vi "Combine I&P.vi"() -> ()   [LabVIEW 2016]
uses:
  <vilib>/userdefined/High Color/IMAQdx.ctl
  <vilib>/vision/driver/NI_Vision_Acquisition_Software.lvlib
panel:
  out "Injector's Position":dbl[](array[numeric])
  in  "sutter run":bool
  in  "Refresh":bool
  out "Cells' pos":dbl[][](array[numeric])
  in  "Cell to Delete":dbl
  in  "stop capture":bool
  out "Image":T1(plugin-control)
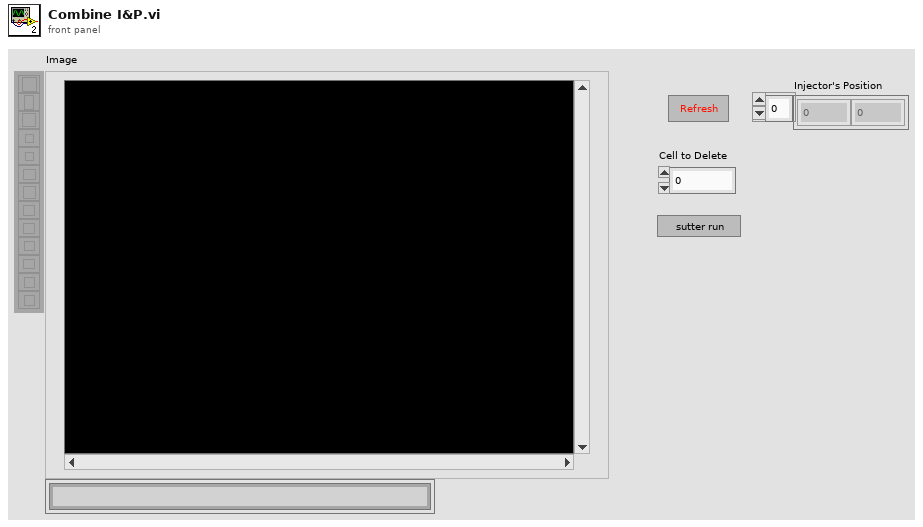
[diagram p1: front panel]
types:
  T1 = typedef "IMAQ Image.ctl" = refnum<image>
  T2 = typedef "IMAQdx.ctl" = refnum<k21>
  T3 = cluster{"Position":cluster{"x":sgl, "y":sgl}, "Angle":sgl, "Scale":sgl, "Score":sgl, "Bounding Box":cluster{"x":sgl, "y":sgl}[]}[]
  T4 = cluster{"Name":string, "Type":enum16{"Line", "Broken Line", "Free Hand Line", "Rotated Rectangle", "Oval", "Polygon", "Free Hand", "Bitmap", "Text"}, "Coordinates":i32[], "Colors":u32[], "Drawing Mode":u32, "Text":string, "Results":cluster{"Process ID":string, "Measure":u16, "Name":string, "String Format":u16, "Width":i16, "Precision":i16, "True String":string, "False String":string}[], "Font, Size & Style":cluster{"Desired Font (Application)":enum16{"User-specified Font", "Application Font", "System Font", "Dialog Font"}, "[User-specified Font]":cluster{"Font Name":string, "Size":i16, "Strikeout?":bool, "Italic?":bool, "Underline?":bool, "Outline?":bool, "Shadow?":bool, "Bold?":bool, "Rotation Angle":dbl}, "Horizontal Alignment":i16, "Vertical Alignment":i16}, "Image File Path":path, "Use Keying Color":bool}[]
  T5 = cluster{"Position":cluster{"x":sgl, "y":sgl}, "Angle":sgl, "Scale":sgl, "Score":sgl, "Bounding Box":cluster{"x":sgl, "y":sgl}[]}
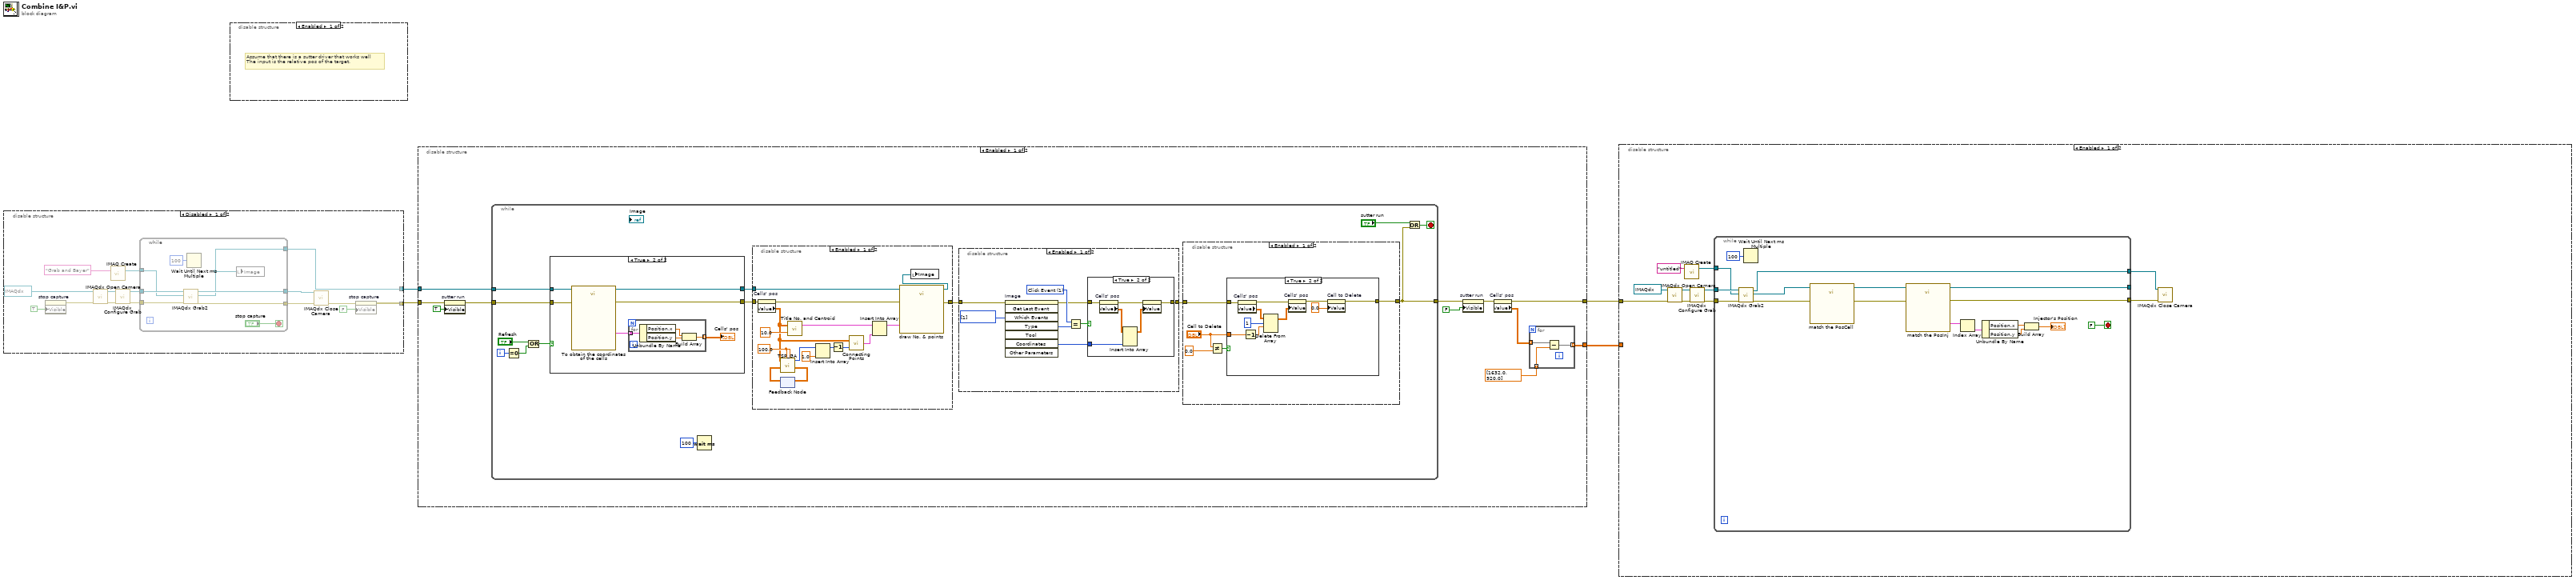
[diagram p0: block diagram]
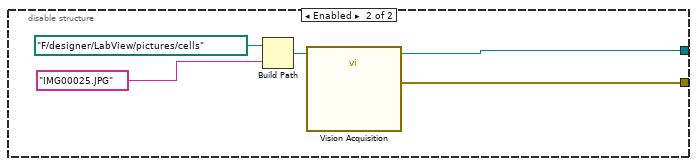
[diagram p11: hidden frame]
diagram:
  n1 = disable-structure shown="Disabled" {
    disable-tunnel: [w5 w28] -> w3
    disable-tunnel: [w19 w29] -> w4
    frame Disabled {
      n2 = property on="stop capture" class="Bool"("Visible"=TRUE) -> (error out=w9:errorcluster)  [unwired: 2 in, 1 out]
      n3 = call <vilib>:"IMAQdx Open Camera.vi"("error in"=w9, "Session In"=T2 "cam0") -> ("error out"=w14:errorcluster, "Session Out"=w15:T2)  [unwired: 1 in, 7 out]
      n4 = call "IMAQ Create"("Image Name"="Grab and Bayer") -> ("New Image"=w12:T1)  [unwired: 3 in, 2 out]
      n5 = call <vilib>:"IMAQdx Configure Grab.vi"("error in"=w14, "Session In"=w15) -> ("error out"=w17:errorcluster, "Session Out"=w16:T2)  [unwired: 8 out]
      n6 = while {
        tunnel: w12 -> [w25]
        tunnel: w17 -> [w26]
        tunnel: w16 -> [w27]
        tunnel: [w24] -> w11
        tunnel: [w23] -> w10
        tunnel: [w20] -> w19
        stop <- "stop capture" stop-if-true
        n7 = call <vilib>:"IMAQdx Grab2.vi"("error in"=w26, "Image In"=w25, "Session In"=w27) -> ("error out"=w23:errorcluster, "Image Out"=w20:T1, "Session Out"=w24:T2)  [unwired: 5 in, 1 out]
        n8 = Wait Until Next ms Multiple(millisecond multiple=u32 100) -> ()  [unwired: 1 out]
        n9 = local write "Image"(w20) -> ()
      }
      n10 = call <vilib>:"IMAQdx Close Camera.vi"("error in"=w10, "Session In"=w11) -> ("error out"=w6:errorcluster)  [unwired: 9 in]
      n11 = property on="stop capture" class="Bool"(error in=w6, "Visible"=FALSE) -> (error out=w5:errorcluster)  [unwired: 1 in, 1 out]
    }
    frame Enabled {
      n12 = Build Path(base path=path "F:/designer/LabView/pictures/cells" ("file path (dialog if empty)"), name or relative path="IMG00025.JPG" ("名称或相对路径")) -> (appended path=w31:path)
      n13 = call "Vision Acquisition"("Image Path"=w31) -> ("Image Out"=w29:T1, "error out"=w28:errorcluster)  [unwired: 25 in]
    }
  }
  n14 = disable-structure shown="Enabled" {
    frame Enabled {
      # "Assume that there is a sutter driver that works well\nThe input is the relative pos of the target."
    }
    frame Disabled {
    }
  }
  n15 = disable-structure shown="Enabled" {
    disable-tunnel: w3 -> [w42 _]
    disable-tunnel: w4 -> [w43 _]
    disable-tunnel: [w34 _] -> w2
    disable-tunnel: [w33 _] -> w1
    frame Enabled {
      n16 = property on="sutter run" class="Bool"(error in=w42, "Visible"=TRUE) -> (error out=w41:errorcluster)  [unwired: 1 in, 1 out]
      n17 = while {
        tunnel: w43 -> [w52]
        tunnel: w41 -> [w60]
        tunnel: [w48] -> w39
        i -> [w57]
        stop <- w47 stop-if-true
        n18 = Equal To 0?(x=w57) -> (x = 0?=w56:bool)
        n19 = Compound Arithmetic op=OR ("复合运算")("Refresh", w56) -> (w59:bool)
        n20 = case shown="True" w59 {
          tunnel: w52 -> [w109 w112]
          tunnel: w60 -> [w110 w116]
          tunnel: [w110 w113] -> w53
          tunnel: [w109 w111] -> w50
          frame False {
          }
          frame True {
            n21 = call "To obtain the coordinates of the cells"("Image In"=w112, "error in"=w116) -> ("Image Out"=w111:T1, "Matches (Color Pattern Matching 1)"=w115:T3, "error out"=w113:errorcluster)  [unwired: 22 in, 1 out]
            n22 = for {
              tunnel: [w119] -> w114 mode=indexing
              tunnel: w115 -> [w120] mode=indexing
              n23 = Unbundle By Name(w120) -> ("Position.x"=w118:sgl, "Position.y"=w117:sgl)
              n24 = Build Array(w118, w117) -> (w119:sgl[])
            }
            "Cells' pos" <- w114
          }
        }
        n25 = Wait (ms)(milliseconds to wait=u32 100 ("等待时间（毫秒）")) -> ()  [unwired: 1 out]
        n26 = disable-structure shown="Enabled" {
          disable-tunnel: w53 -> [w77 _]
          disable-tunnel: [w74 _] -> w51
          disable-tunnel: w50 -> [w73 _]
          frame Enabled {
            w69 = 100.0 ("pop_size")
            n27 = property on="Cells' pos" class="Arr (strict)"(error in=w77) -> (error out=w75:errorcluster, "Value"=w68:dbl[][])  [unwired: 1 in, 1 out]
            n28 = feedback #1() -> (w70:dbl[][])  [unwired: 1 in]
            n29 = call "TSP_GA.vi"("Number of Iterative"=w69, "pop_size"=w69, "Pop in"=w70, "xy"=w68) -> ("pop out"=w71:dbl[][], "opt_rte"=w62:i16[])  [unwired: 3 in, 3 out]
            n30 = feedback-in #1(w71) -> ()
            n31 = call "Title No. and Centroid.vi"("半径"=10.0, "Particle Measurements (Pixels)"=w68) -> ("输出数组"=w67:T4)  [unwired: 1 out]
            n32 = Insert Into Array(array=w62, new element=1.0 ("element")) -> (w63:i16[])  [unwired: 1 in]
            n33 = Decrement(x=w63) -> (x-1=w61:i16[])
            n34 = call "Connecting Points.vi"("index"=w61, "数组"=w68) -> ("输出数组"=w65:T4)
            n35 = Insert Into Array(array=w67, new element=w65) -> (w66:T4)  [unwired: 1 in]
            n36 = call "draw No. & points"("Image In"=w73, "Parameters (Overlay 1)"=w66, "error in"=w75) -> ("Image Out"=w76:T1, "error out"=w74:errorcluster)  [unwired: 23 in]
            n37 = local write "Image"(w76) -> ()
          }
          frame Disabled {
          }
        }
        n38 = disable-structure shown="Enabled" {
          disable-tunnel: [w79 _] -> w54
          disable-tunnel: w51 -> [w78 _]
          frame Enabled {
            w83 = 1 items=["No Event"=0, "Click Event"=1, "Draw Event"=2, "Size Event"=4, "Scroll Event"=5, "Double Click Event"=8]
            w84 = i32[] [1] items=["No Event"=0, "Click Event"=1, "Draw Event"=2, "Size Event"=4, "Scroll Event"=5, "Double Click Event"=8] ("Which Events")
            n39 = invoke on="Image" class="ImageControl" method="Get Last Event"(error in=w78, "Which Events"=w84) -> (error out=w80:errorcluster, "Type"=w82:i32, "Coordinates"=w85:i32[])  [unwired: 6 in, 5 out]
            n40 = Equal?(x=w83, y=w82) -> (x = y?=w81:bool)
            n41 = case shown="True" w81 {
              tunnel: w85 -> [_ w92]
              tunnel: w80 -> [w86 w89]
              tunnel: [w86 w87] -> w79
              frame False {
              }
              frame True {
                n42 = property on="Cells' pos" class="Arr (strict)"(error in=w89) -> (error out=w88:errorcluster, "Value"=w91:dbl[][])  [unwired: 1 in, 1 out]
                n43 = Insert Into Array(array=w91, new element=w92) -> (w90:dbl[][])  [unwired: 2 in]
                n44 = property on="Cells' pos" class="Arr (strict)"(error in=w88, "Value"=w90) -> (error out=w87:errorcluster)  [unwired: 1 in, 1 out]
              }
            }
          }
          frame Disabled {
          }
        }
        n45 = disable-structure shown="Enabled" {
          disable-tunnel: w54 -> [w97 _]
          disable-tunnel: [w93 _] -> w48
          frame Enabled {
            n46 = Not Equal?(x="Cell to Delete", y=0.0) -> (x != y?=w95:bool)
            n47 = case shown="True" w95 {
              tunnel: "Cell to Delete" -> [_ w106]
              tunnel: w97 -> [w98 w100]
              tunnel: [w98 w99] -> w93
              frame False {
              }
              frame True {
                n48 = property on="Cells' pos" class="Arr (strict)"(error in=w100) -> (error out=w102:errorcluster, "Value"=w105:dbl[][])  [unwired: 1 in, 1 out]
                n49 = Decrement(x=w106) -> (x-1=w107:dbl)
                n50 = Delete From Array(array=w105, length=1 ("长度"), index (row)=w107) -> (array with subset deleted=w104:dbl[][])  [unwired: 1 in, 1 out]
                n51 = property on="Cells' pos" class="Arr (strict)"(error in=w102, "Value"=w104) -> (error out=w101:errorcluster)  [unwired: 1 in, 1 out]
                n52 = property on="Cell to Delete" class="DigNum (strict)"(error in=w101, "Value"=0.0 ("细胞序号")) -> (error out=w99:errorcluster)  [unwired: 1 in, 1 out]
              }
            }
          }
          frame Disabled {
          }
        }
        n53 = Or(x="sutter run", y=w48) -> (x .or. y?=w47:bool)
      }
      n54 = property on="sutter run" class="Bool"(error in=w39, "Visible"=FALSE) -> (error out=w37:errorcluster)  [unwired: 1 in, 1 out]
      n55 = property on="Cells' pos" class="Arr (strict)"(error in=w37) -> (error out=w33:errorcluster, "Value"=w36:dbl[][])  [unwired: 1 in, 1 out]
      n56 = for {
        tunnel: w36 -> [w46] mode=indexing
        tunnel: dbl[] [1632.0, 920.0] ("Value") -> [w45] mode=indexing
        tunnel: [w44] -> w34 mode=indexing
        n57 = Subtract(x=w46, y=w45) -> (x-y=w44:dbl[])
      }
    }
    frame Disabled {
    }
  }
  n58 = disable-structure shown="Enabled" {
    disable-tunnel: w2 -> [_ _]
    disable-tunnel: w1 -> [w123 _]
    frame Enabled {
      n59 = call <vilib>:"IMAQdx Open Camera.vi"("error in"=w123, "Session In"=T2 "cam0") -> ("error out"=w128:errorcluster, "Session Out"=w127:T2)  [unwired: 1 in, 7 out]
      n60 = call "IMAQ Create"("Image Name"="untitled") -> ("New Image"=w129:T1)  [unwired: 3 in, 2 out]
      n61 = call <vilib>:"IMAQdx Configure Grab.vi"("error in"=w128, "Session In"=w127) -> ("error out"=w125:errorcluster, "Session Out"=w126:T2)  [unwired: 8 out]
      n62 = while {
        tunnel: w129 -> [w145]
        tunnel: w125 -> [w146]
        tunnel: w126 -> [w147]
        tunnel: [w137] -> _
        tunnel: [w136] -> w130
        tunnel: [w140] -> w121
        stop <- FALSE stop-if-true
        n63 = call <vilib>:"IMAQdx Grab2.vi"("error in"=w146, "Image In"=w145, "Session In"=w147) -> ("error out"=w142:errorcluster, "Image Out"=w141:T1, "Session Out"=w140:T2)  [unwired: 5 in, 1 out]
        n64 = Wait Until Next ms Multiple(millisecond multiple=u32 100) -> ()  [unwired: 1 out]
        n65 = call "match the PosCell"("Image In"=w141, "error in"=w142) -> ("Image Out"=w139:T1, "error out"=w138:errorcluster)  [unwired: 24 in]
        n66 = call "match the PosInj"("Image In"=w139, "error in"=w138) -> ("Image Out"=w137:T1, "Matches (Pattern Matching 1)"=w133:T3, "error out"=w136:errorcluster)  [unwired: 23 in]
        n67 = Index Array(array=w133) -> (element=w132:T5)  [unwired: 1 in]
        n68 = Unbundle By Name(w132) -> ("Position.x"=w135:sgl, "Position.y"=w134:sgl)
        n69 = Build Array(w135, w134) -> (→"Injector's Position":sgl[])
      }
      n70 = call <vilib>:"IMAQdx Close Camera.vi"("error in"=w130, "Session In"=w121) -> ()  [unwired: 9 in, 1 out]
    }
    frame Disabled {
    }
  }
